vi "Add Tasks.vi"(8 "error in (no error)":errorcluster, 10 "User Selections":string[](array[string]), 11 "BuildServer in":refnum<class "BuildServer.lvclass">) -> (0 "error out":errorcluster, 3 "BuildServer out":refnum<class "BuildServer.lvclass">)   [LabVIEW 2017, in "BuildServer.lvlib" / "BuildServer.lvclass"]
uses:
  BuildServer.lvclass
  C:/Program Files (x86)/National Instruments/LabVIEW 2017/vi.lib/ActorFramework/Actor/Actor.lvclass
  <vilib>/ActorFramework/Actor/Actor.lvclass/Actor.ctl
  <vilib>/ActorFramework/Message Enqueuer/Message Enqueuer.lvclass/Message Enqueuer.ctl
  <vilib>/ActorFramework/Message Enqueuer/Init from Existing Queue.vi
  <vilib>/ActorFramework/Message Enqueuer/Enqueue.vi
  BuildServer Messages/Update TaskView Msg/Update TaskView Msg.lvclass
  C:/Program Files (x86)/National Instruments/LabVIEW 2017/vi.lib/ActorFramework/Message/Message.lvclass
  <vilib>/ActorFramework/Message Priority Queue/Priority Enqueue.vi
  <vilib>/ActorFramework/Message Enqueuer/Message Enqueuer.lvclass
  <vilib>/ActorFramework/Actor/Actor.lvclass
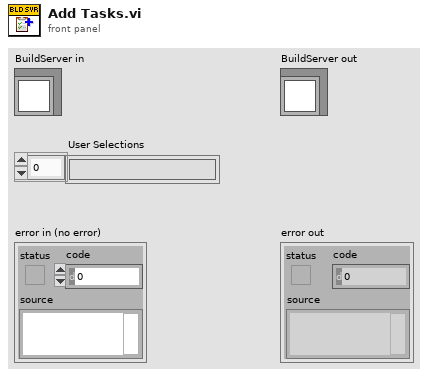
[diagram p1: front panel]
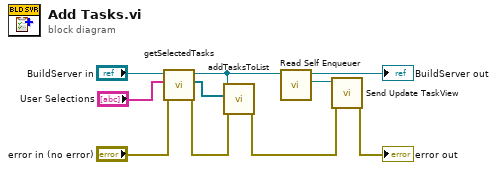
[diagram p0: block diagram]
diagram:
  n1 = call "getSelectedTasks.vi"("error in (no error)"="error in (no error)", "User Selections"="User Selections", "BuildServer in"="BuildServer in") -> ("error out"=w5:errorcluster, "Selected Tasks"=w6:refnum<class "Task.lvclass">[], "BuildServer out"=w4:refnum<class "BuildServer.lvclass">)  [unwired: 6 in]
  "BuildServer out" <- w4
  n2 = call "addTasksToList.vi"("error in (no error)"=w5, "Selected Tasks"=w6, "BuildServer in"=w4) -> ("error out"=w2:errorcluster)  [unwired: 8 in]
  n3 = call <vilib>:"Read Self Enqueuer.vi"("Actor"=w4) -> ("Self Enqueuer"=w3:refnum<class "Message Enqueuer.lvclass">)  [unwired: 10 in]
  n4 = call "Send Update TaskView.vi"("error in (no error)"=w2, "Message Enqueuer in"=w3) -> ("error out"=→"error out":errorcluster)  [unwired: 8 in, 1 out]
